vi "Test.vi"() -> ()   [LabVIEW 2014, in "Analyze.lvlib" / "Analyze Fluence.lvclass"]
uses:
  Analyze Fluence.lvclass
panel:
  out "error out":errorcluster
  in  "Origin":cluster{"X":i32, "Y":i32}
  in  "String":string
  in  "error in (no error)":errorcluster
  in  "Font, Size & Style":T1={"Desired Font (Application)"=enum."Application Font", "[User-specified Font]"={"Font Name"="", "Size"=12, "Strikeout?"=FALSE, "Italic?"=FALSE, "Underline?"=FALSE, "Outline?"=FALSE, "Shadow?"=FALSE, "Bold?"=FALSE, "Rotation Angle"=0.0}, "Horizontal Alignment"=0, "Vertical Alignment"=0} {"Vertical Alignment" items=["Bottom", "Top", "Baseline"]; "Horizontal Alignment" items=["Left", "Center", "Right"]; "[User-specified Font]"."Rotation Angle" format="%.2f"}
  in  "Text Color (black)":u32(colorbox)
  in  "BG Color (Transparent)":u32(colorbox)=16777216
  out "Counts in Tiles 2":i64[][](array[numeric])
  out "Maximum":i64
  out "Max Index":i32[](array[numeric])
  out "max index(es)":i32[](array[numeric])
  out "max value":i64
  out "Counts in Tiles":i64[][](array[numeric])
  out "Image":T2(plugin-control)
  in  "size":i32
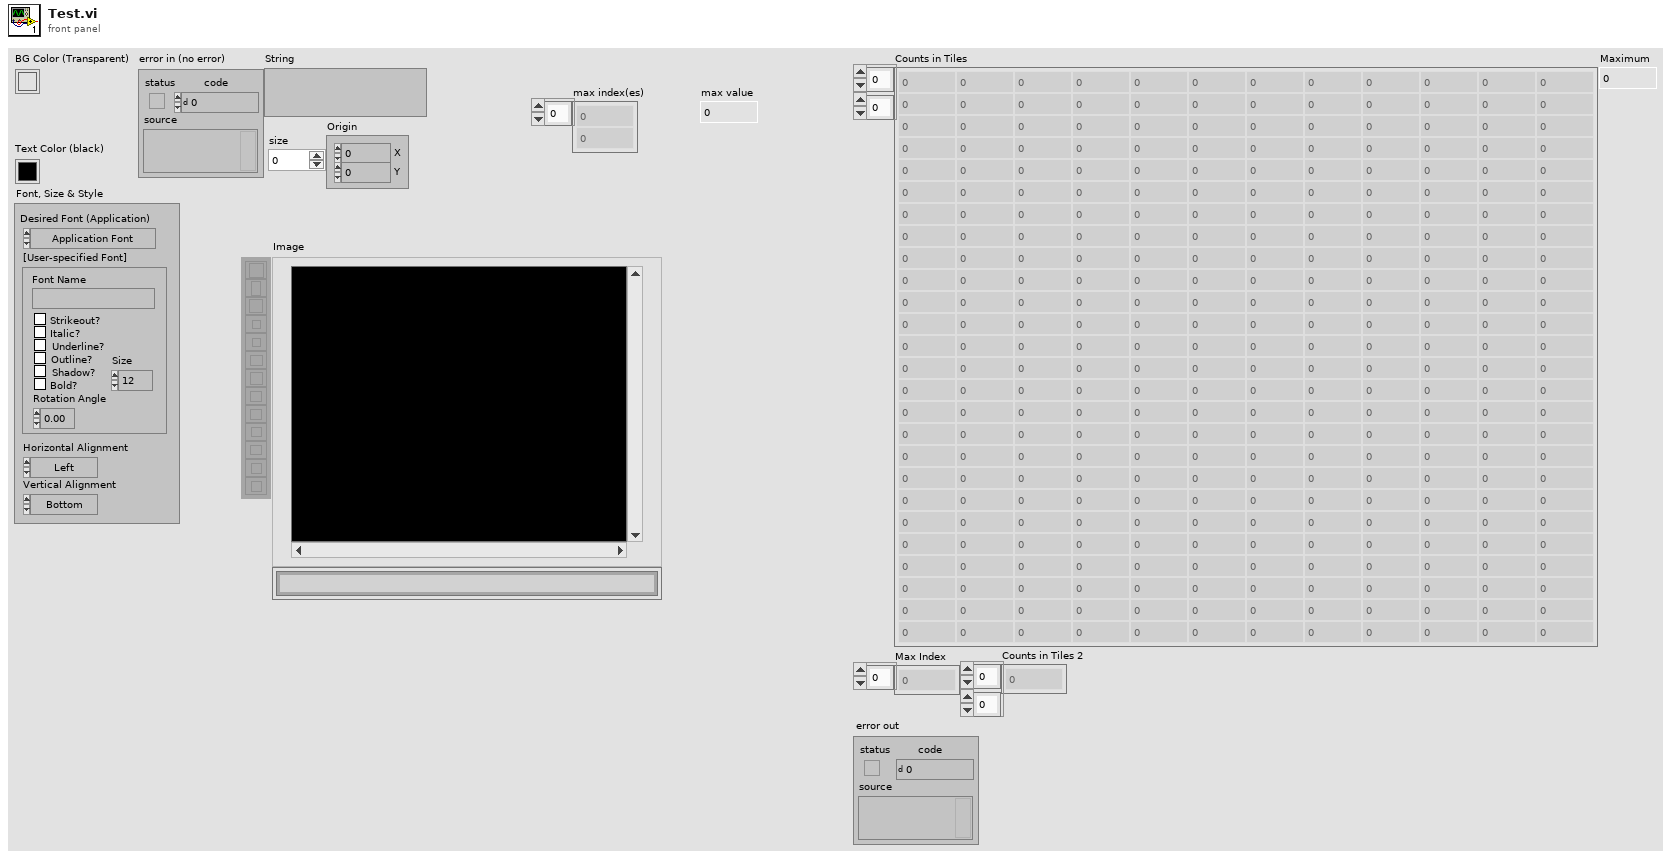
[diagram p1: front panel]
types:
  T1 = cluster{"Desired Font (Application)":enum16{"User-specified Font", "Application Font", "System Font", "Dialog Font"}, "[User-specified Font]":cluster{"Font Name":string, "Size":i16, "Strikeout?":bool, "Italic?":bool, "Underline?":bool, "Outline?":bool, "Shadow?":bool, "Bold?":bool, "Rotation Angle":dbl}, "Horizontal Alignment":i16, "Vertical Alignment":i16}
  T2 = typedef "IMAQ Image.ctl" = refnum<image>
  T3 = typedef "Image Type" = u32
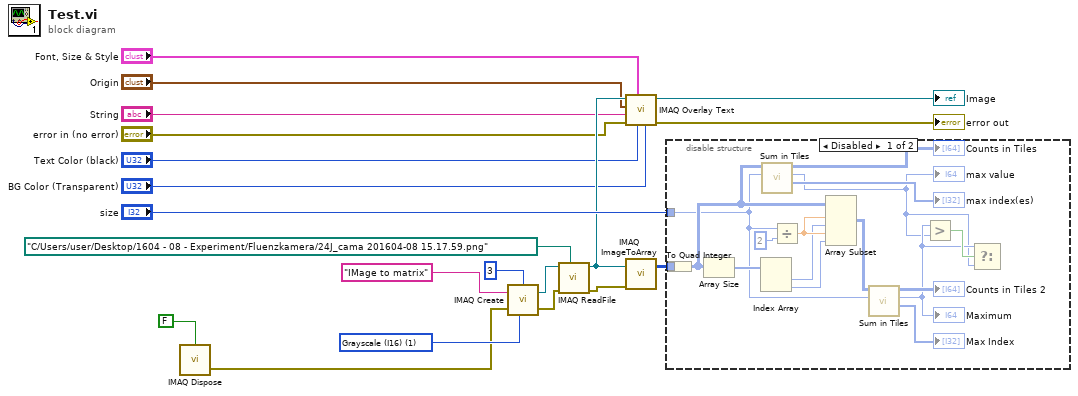
[diagram p0: block diagram]
diagram:
  w15 = T3 1 items=["Grayscale (U8)", "Grayscale (I16)", "Grayscale (SGL)", "Complex (CSG)", "RGB (U32)", "HSL (U32)", "RGB (U64)", "Grayscale (U16)"] ("Image Type")
  n1 = call "IMAQ Dispose"("All Images? (No)"=FALSE) -> ("error out"=w1:errorcluster)  [unwired: 5 in]
  n2 = call "IMAQ Create"("Border Size"=3, "Image Name"="IMage to matrix", "Image Type"=w15, "error in (no error)"=w1) -> ("New Image"=w19:T2, "error out"=w17:errorcluster)  [unwired: 1 in]
  n3 = call "IMAQ ReadFile"("File Path"=path "C:/Users/user/Desktop/1604 - 08 - Experiment/Fluenzkamera/24J_cama 201604-08 15.17.59.png", "error in (no error)"=w17, "Image"=w19) -> ("error out"=w14:errorcluster, "Image Out"=w11:T2)  [unwired: 4 in, 3 out]
  n4 = call "IMAQ Overlay Text"("BG Color (Transparent)"="BG Color (Transparent)", "Text Color (black)"="Text Color (black)", "Font, Size & Style"="Font, Size & Style", "error in (no error)"="error in (no error)", "String"="String", "Origin"="Origin", "Image"=w11) -> ("error out"=→"error out":errorcluster, "Image Out"=→"Image":T2)  [unwired: 3 in]
  n5 = call "IMAQ ImageToArray"("error in (no error)"=w14, "Image"=w11) -> ("Image Pixels (I16)"=w13:i16[][])  [unwired: 2 in, 4 out]
  n6 = disable-structure shown="Disabled" {
    disable-tunnel: w13 -> [w36 _]
    disable-tunnel: "size" -> [w26 _]
    frame Disabled {
      n7 = To Quad Integer(1:w36) -> (0:w31:i64[][])
      n8 = Array Size(array=w31) -> (size(s)=w30:i32[])
      n9 = Index Array(array=w30) -> (element #1=w29:i32, element #2=w28:i32)  [unwired: 2 in]
      n10 = call "Sum in Tiles.vi"("size"=w26, "Image"=w31) -> ("Max Index"=→"max index(es)":i32[], "Maximum"=w21:i64, "Counts in Tiles"=→"Counts in Tiles":i64[][])  [unwired: 7 in]
      "max value" <- w21
      n11 = Divide(x=w26, y=2 ("x")) -> (x/y=w32:dbl)
      n12 = Array Subset(array=w31, index (row)=w32, length (row)=w29, index (col)=w32, length (col)=w28) -> (w27:i64[][])
      n13 = call "Sum in Tiles.vi"("size"=w26, "Image"=w27) -> ("Max Index"=→"Max Index":i32[], "Maximum"=w22:i64, "Counts in Tiles"=→"Counts in Tiles 2":i64[][])  [unwired: 7 in]
      "Maximum" <- w22
      n14 = Greater?(x=w22, y=w21) -> (0:w23:bool)
      n15 = Select(t=w22, s=w23, f=w21) -> ()  [unwired: 1 out]
    }
    frame Enabled {
    }
  }
